vi "probe device.vi"(8 "error in (no error)":errorcluster, 11 "uri":string) -> (0 "error out":errorcluster, 3 "function return":i32)   [LabVIEW 2012, in "libximc.lvlib"]
doc: "result_t XIMC_API probe_device (const char* uri);"
uses:
  libximc.lvlib
  libximc.dll
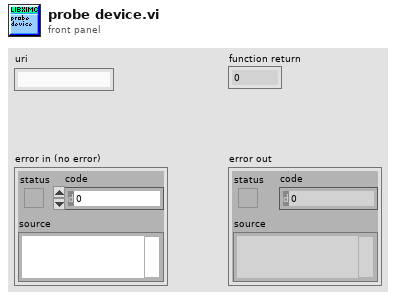
[diagram p1: front panel]
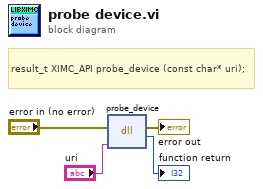
[diagram p0: block diagram]
diagram:
  # "result_t XIMC_API probe_device (const char* uri);"
  n1 = dll-call lib="E:/labview-2.12.1-Labview_12.0/ximcLVx32/libximc.*" fn="probe_device"(error in="error in (no error)", "uri"="uri") -> (error out=→"error out":errorcluster, →"function return":i32)  [unwired: 3 in, 1 out]
